vi "subViFormulaGenerator_4pulse.vi"(0 "offset":dbl format="%0.2p", 1 "sampling info":cluster{"Fs":dbl, "#s":dbl}={"Fs"=1000.0, "#s"=1000.0} {"Fs" format="%.2p"}, 2 "scale":dbl=1.0 format="%0.2f", 3 "error in (no error)":errorcluster, 4 "functionInfo":T1={"time1"=0.0, "formula1"="0", "time2"=0.0, "formula2"="0", "time3"=0.0, "formula3"="0", "time4"=0.0, "formula4"="0"}) -> (5 "waveform out":waveform(dbl), 6 "error out":errorcluster)   [LabVIEW 2021]
uses:
  <vilib>/Waveform/WDTOps.llb/WDT Append Waveforms DBL.vi
  <vilib>/measure/NI_MAPro.lvlib
panel:
  # "子程序，用于产生一个四段的分段函数，根据板卡的特性可以调节函数的offset和scale"
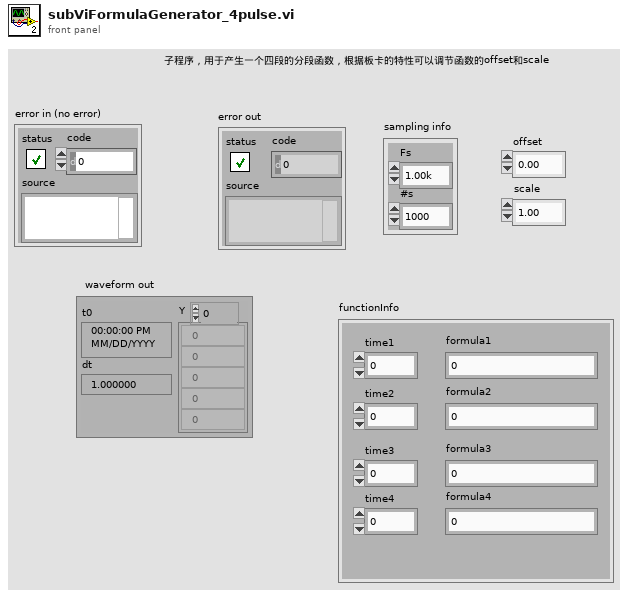
[diagram p1: front panel]
types:
  T1 = cluster{"time1":dbl, "formula1":string, "time2":dbl, "formula2":string, "time3":dbl, "formula3":string, "time4":dbl, "formula4":string}
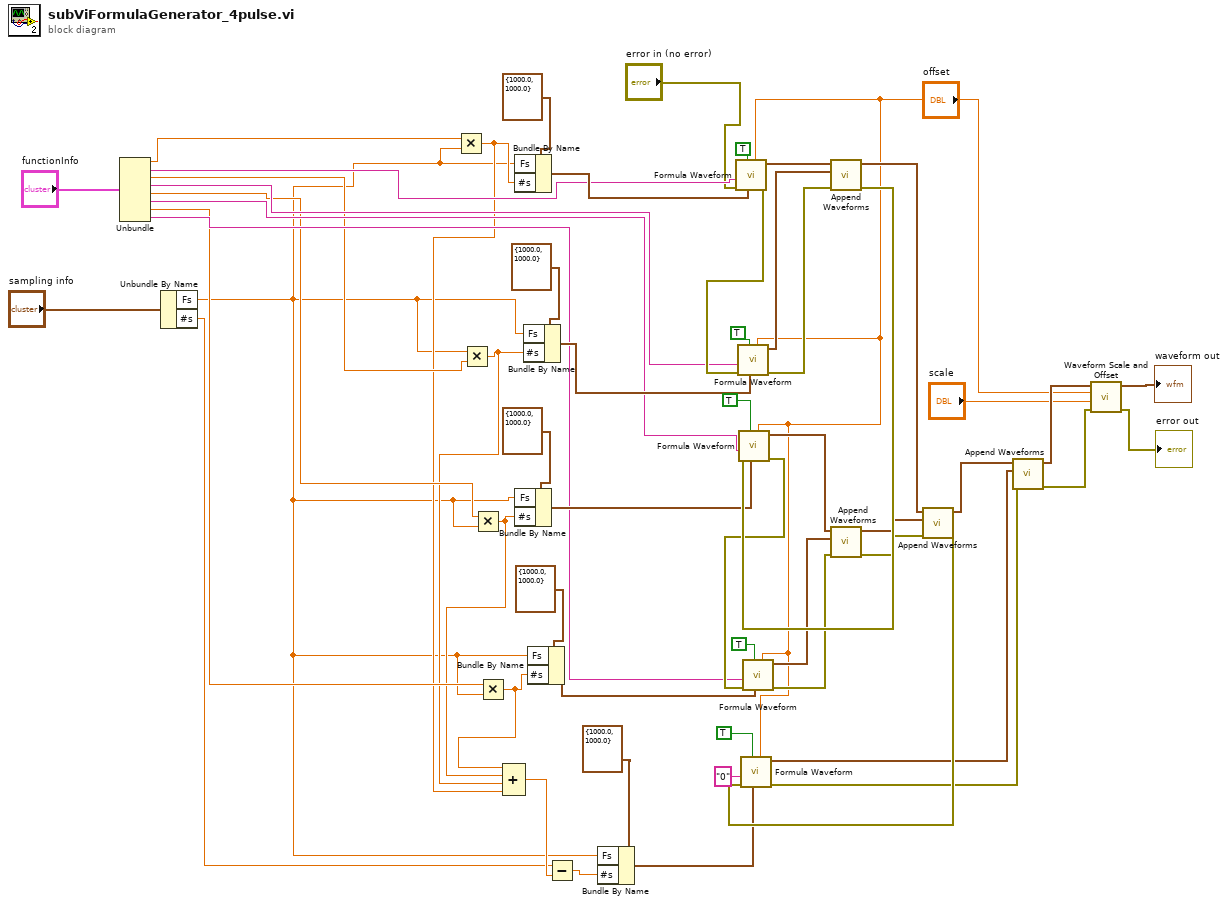
[diagram p0: block diagram]
diagram:
  n1 = Unbundle("functionInfo") -> ("time1"=w25:dbl, "formula1"=w29:string, "time2"=w24:dbl, "formula2"=w32:string, "time3"=w23:dbl, "formula3"=w31:string, "time4"=w22:dbl, "formula4"=w30:string)
  n2 = Unbundle By Name("sampling info") -> ("Fs"=w5:dbl, "#s"=w7:dbl)
  n3 = Multiply(x=w25, y=w5) -> (x*y=w12:dbl)
  n4 = Multiply(x=w5, y=w24) -> (x*y=w11:dbl)
  n5 = Multiply(x=w23, y=w5) -> (x*y=w10:dbl)
  n6 = Multiply(x=w22, y=w5) -> (x*y=w9:dbl)
  n7 = Compound Arithmetic op=ADD(w9, w10, w11, w12) -> (w8:dbl)
  n8 = Bundle By Name(cluster=cluster{"Fs":dbl, "#s":dbl} {"Fs"=1000.0, "#s"=1000.0} ("sampling info"), "Fs"=w5, "#s"=w12) -> (w47:cluster{"Fs":dbl, "#s":dbl})
  n9 = Bundle By Name(cluster=cluster{"Fs":dbl, "#s":dbl} {"Fs"=1000.0, "#s"=1000.0} ("sampling info"), "Fs"=w5, "#s"=w10) -> (w45:cluster{"Fs":dbl, "#s":dbl})
  n10 = Bundle By Name(cluster=cluster{"Fs":dbl, "#s":dbl} {"Fs"=1000.0, "#s"=1000.0} ("sampling info"), "Fs"=w5, "#s"=w11) -> (w43:cluster{"Fs":dbl, "#s":dbl})
  n11 = Bundle By Name(cluster=cluster{"Fs":dbl, "#s":dbl} {"Fs"=1000.0, "#s"=1000.0} ("sampling info"), "Fs"=w5, "#s"=w9) -> (w26:cluster{"Fs":dbl, "#s":dbl})
  n12 = Subtract(x=w7, y=w8) -> (x-y=w6:dbl)
  n13 = Bundle By Name(cluster=cluster{"Fs":dbl, "#s":dbl} {"Fs"=1000.0, "#s"=1000.0} ("sampling info"), "Fs"=w5, "#s"=w6) -> (w4:cluster{"Fs":dbl, "#s":dbl})
  n14 = call <vilib>:"Formula Waveform.vi"("offset"="offset", "sampling info"=w47, "reset signal"=TRUE, "error in (no error)"="error in (no error)", "formula"=w29) -> ("error out"=w54:errorcluster, "signal out"=w53:waveform(dbl))  [unwired: 5 in]
  n15 = call <vilib>:"Formula Waveform.vi"("offset"="offset", "sampling info"=w43, "reset signal"=TRUE, "error in (no error)"=w54, "formula"=w32) -> ("error out"=w51:errorcluster, "signal out"=w52:waveform(dbl))  [unwired: 5 in]
  n16 = call-poly <vilib>:"Append Waveforms.vi"("error in (no error)"=w51, "waveform B"=w52, "waveform A"=w53) -> ("error out"=w50:errorcluster, "waveform out"=w49:waveform(dbl))  [unwired: 7 in]
  n17 = call <vilib>:"Formula Waveform.vi"("offset"="offset", "sampling info"=w45, "reset signal"=TRUE, "error in (no error)"=w50, "formula"=w31) -> ("error out"=w39:errorcluster, "signal out"=w40:waveform(dbl))  [unwired: 5 in]
  n18 = call <vilib>:"Formula Waveform.vi"("offset"="offset", "sampling info"=w26, "reset signal"=TRUE, "error in (no error)"=w39, "formula"=w30) -> ("error out"=w37:errorcluster, "signal out"=w38:waveform(dbl))  [unwired: 5 in]
  n19 = call-poly <vilib>:"Append Waveforms.vi"("error in (no error)"=w37, "waveform B"=w38, "waveform A"=w40) -> ("error out"=w35:errorcluster, "waveform out"=w34:waveform(dbl))  [unwired: 7 in]
  n20 = call-poly <vilib>:"Append Waveforms.vi"("error in (no error)"=w35, "waveform B"=w34, "waveform A"=w49) -> ("error out"=w21:errorcluster, "waveform out"=w16:waveform(dbl))  [unwired: 7 in]
  n21 = call <vilib>:"Formula Waveform.vi"("offset"="offset", "sampling info"=w4, "reset signal"=TRUE, "error in (no error)"=w21, "formula"="0") -> ("error out"=w14:errorcluster, "signal out"=w17:waveform(dbl))  [unwired: 5 in]
  n22 = call-poly <vilib>:"Append Waveforms.vi"("error in (no error)"=w14, "waveform B"=w17, "waveform A"=w16) -> ("error out"=w13:errorcluster, "waveform out"=w15:waveform(dbl))  [unwired: 7 in]
  n23 = call <vilib>:"Waveform Scale and Offset.vi"("error in (no error)"=w13, "scale"="scale", "offset"="offset", "waveform in"=w15) -> ("error out"=→"error out":errorcluster, "waveform out"=→"waveform out":waveform(dbl))  [unwired: 6 in]
